vi "Get Data.vi"(11 "Static Path Selector in":refnum<class "MGI Static Path Selector.lvclass">) -> (2 "Persistent":T1={"Path"=path "", "Select Option?"=TRUE, "Explorer Option?"=TRUE, "Recurse?"=TRUE, "Allow New?"=FALSE, "Filter"="*.*"})   [LabVIEW 2016, in "MGI Static Path Selector.lvclass"]
doc: "Sets the private data as specified."
uses:
  <userlib>/_MGI/User Interface/Path Selector XControl/Class Hierarchy/Static File Selector/MGI Static Path Selector.lvclass
  <userlib>/_MGI/User Interface/Path Selector XControl/Class Hierarchy/Static File Selector/Persistent Data Cluster.ctl
  <userlib>/_MGI/User Interface/Path Selector XControl/Class Hierarchy/Static File Selector/MGI Static Path Selector.lvclass/MGI Static Path Selector.ctl
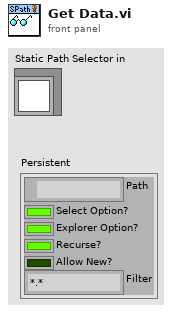
[diagram p1: front panel]
types:
  T1 = typedef "MGI Static Path Selector.lvclass/Persistent Data Cluster.ctl" = cluster{"Path":path, "Select Option?":bool, "Explorer Option?":bool, "Recurse?":bool, "Allow New?":bool, "Filter":string}
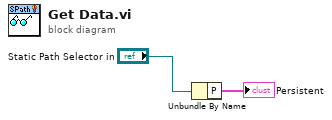
[diagram p0: block diagram]
diagram:
  n1 = Unbundle By Name("Static Path Selector in") -> ("P"=→"Persistent":T1)
